vi "Construct.vi"(6 "Delimiter (,)":string=",", 8 "error in (no error)":errorcluster, 10 "Headers[]":string[](array[string]), 11 "File Path":path) -> (0 "error out":errorcluster, 3 "SLL CSV Logger out":refnum<class "SLL CSV Logger.lvclass">)   [LabVIEW 2014, in "SLL Spreadsheet.lvlib" / "SLL CSV Logger.lvclass"]
doc: "Constructs the CSV Logger Object with the logger path, delimiter and the initial header list. \n\nThe header list is optional. New headers can be dynamically added during logging as well."
uses:
  SLL CSV Logger.lvclass
  SLL CSV Logger.lvclass/SLL CSV Logger.ctl
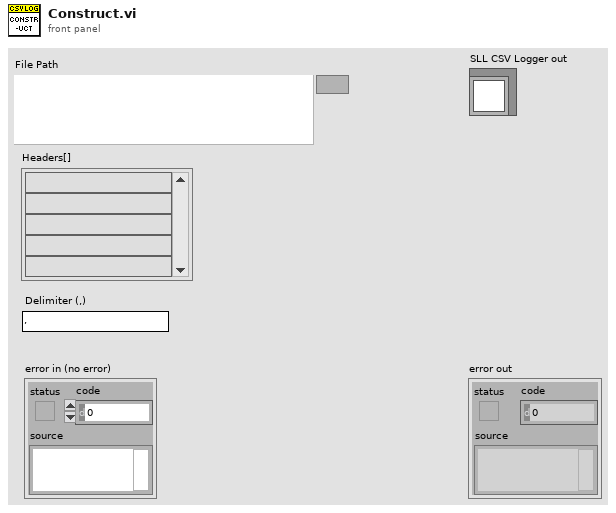
[diagram p1: front panel]
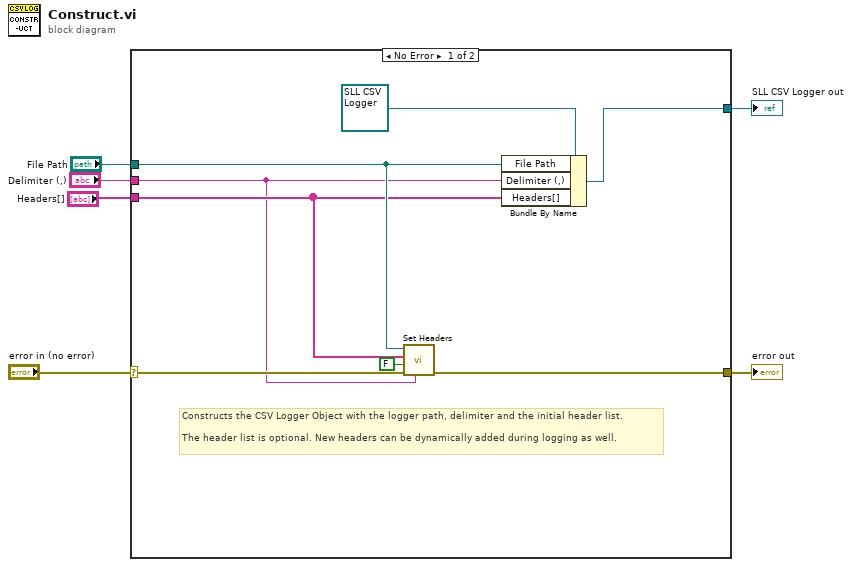
[diagram p0: block diagram]
diagram:
  n1 = case shown="No Error" "error in (no error)" {
    selector: "error in (no error)" -> [w12 w15]
    tunnel: [w11 w15] -> w5
    tunnel: [w13 _] -> w4
    tunnel: "File Path" -> [w10 _]
    tunnel: "Delimiter (,)" -> [w8 _]
    tunnel: "Headers[]" -> [w9 _]
    frame No Error {
      # "Constructs the CSV Logger Object with the logger path, delimiter and the initial header list. \n\nThe header list is optional. New headers can be dynamically added during logging as well."
      n2 = call "Set Headers.vi"("Delimiter (,)"=w8, "error in (no error)"=w12, "Update Existing? (T)"=FALSE ("Update Existing? (F)"), "Headers[]"=w9, "File Path"=w10) -> ("error out"=w11:errorcluster)  [unwired: 5 in, 1 out]
      n3 = Bundle By Name(cluster=refnum<class "SLL CSV Logger.lvclass"> refnum ("SLL Spreadsheet Logger in"), "File Path"=w10, "Delimiter (,)"=w8, "Headers[]"=w9) -> (w13:refnum<class "SLL CSV Logger.lvclass">)
    }
    frame Error {
    }
  }
  "error out" <- w5
  "SLL CSV Logger out" <- w4
